vi "ParseSerializableClassHeader.vi"(8 "error in (no error)":errorcluster, 10 "Version":string[](array[string]), 11 "Class":string[](array[string])) -> (0 "error out":errorcluster, 3 "SerializedClassHeader (child,parent)":T1[](array[typedef]))   [LabVIEW 2019, in "BlueSerialization.lvlib" / "BlueSerializer.lvclass"]
uses:
  BlueSerializer.lvclass
  ClassHeader.ctl
  <vilib>/Utility/EditLVLibs/LibVersion.ctl
  <vilib>/Utility/error.llb/Error Cluster From Error Code.vi
  <vilib>/Utility/LVClass/Get LV Class Name.vi
  <vilib>/ErrorRing/Error Ring.xnode
  BlueSerializable/BlueSerializable.lvclass
  <vilib>/Utility/EditLVLibs/Edit LVLibs.lvlib
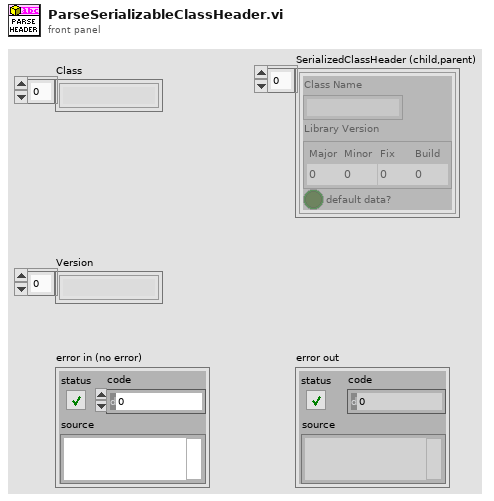
[diagram p1: front panel]
types:
  T1 = typedef "BlueSerialization.lvlib/BlueSerializer.lvclass/ClassHeader.ctl" = cluster{"Class Name":string, "Library Version":T2, "default data?":bool}
  T2 = typedef "Edit LVLibs.lvlib/LibVersion.ctl" = cluster{"Major":u16, "Minor":u16, "Fix":u16, "Build":u16}
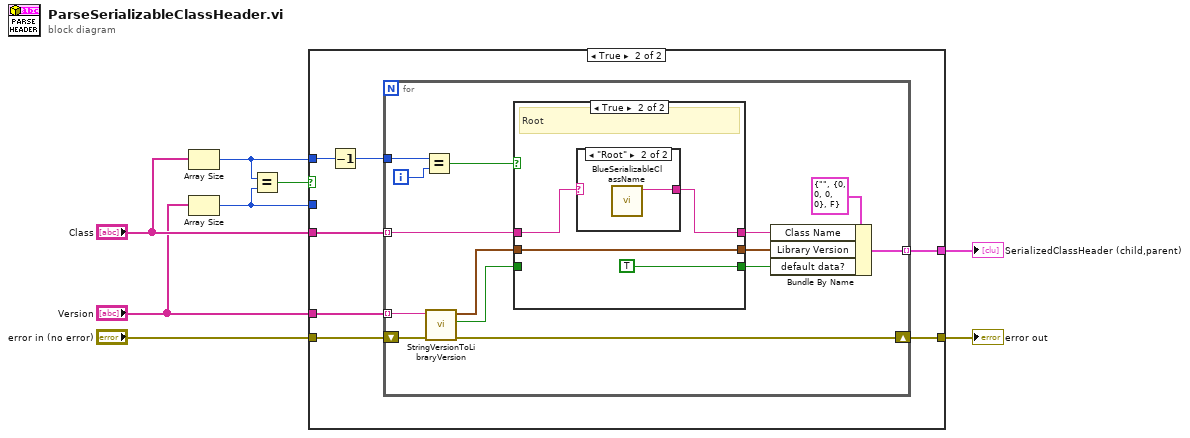
[diagram p0: block diagram]
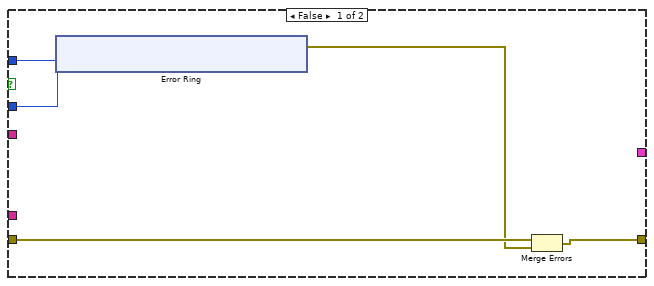
[diagram p2: hidden frame]
diagram:
  n1 = Array Size(array="Class") -> (size(s)=w3:i32)
  n2 = Array Size(array="Version") -> (size(s)=w2:i32)
  n3 = Equal?(x=w3, y=w2) -> (x = y?=w8:bool)
  n4 = case shown="True" w8 {
    tunnel: "Class" -> [_ w22]
    tunnel: "Version" -> [_ w28]
    tunnel: "error in (no error)" -> [w11 w27]
    tunnel: [w9 w26] -> w4
    tunnel: w3 -> [w13 w24]
    tunnel: w2 -> [w12 _]
    tunnel: [_ w25] -> w1
    frame False {
      n5 = xnode "Error Ring"("parameter 0"=w13, "parameter 1"=w12) -> ("error out"=w10:errorcluster)
      n6 = Merge Errors(w11, w10) -> (w9:errorcluster)
    }
    frame True {
      n7 = Decrement(x=w24) -> (x-1=w23:i32)
      n8 = for {
        tunnel: w28 -> [w41] mode=indexing
        shift-right: [w39] -> w26
        shift-left: w27 -> [w40]
        tunnel: [w38] -> w25 mode=indexing
        tunnel: w23 -> [w37]
        tunnel: w22 -> [w29] mode=indexing
        i -> [w36]
        n9 = Equal?(x=w37, y=w36) -> (x = y?=w35:bool)
        n10 = call "StringVersionToLibraryVersion.vi"("error in (no error)"=w40, "Version (as serialized)"=w41) -> ("error out"=w39:errorcluster, "default data?"=w32:bool, "Library Version"=w34:T2)  [unwired: 7 in]
        n11 = case shown="True" w35 {
          tunnel: w34 -> [w45 w47]
          tunnel: [w45 w47] -> w33
          tunnel: w32 -> [w44 _]
          tunnel: [w44 TRUE ("default data?")] -> w31
          tunnel: [w43 w48] -> w30
          tunnel: w29 -> [w43 w49]
          frame False {
            # "not root"
          }
          frame True {
            # "Root"
            n12 = case shown="\"Root\"" w49 {
              selector: w49 -> [w50 _]
              tunnel: [w50 w51] -> w48
              frame Default {
              }
              frame "Root" {
                n13 = call "BlueSerializableClassName.vi"() -> ("BlueSerialization.lvlib:BlueSerializable.lvclass"=w51:string)  [unwired: 11 in]
              }
            }
          }
        }
        n14 = Bundle By Name(cluster=T1 {"Class Name"="", "Library Version"={"Major"=0, "Minor"=0, "Fix"=0, "Build"=0}, "default data?"=FALSE} ("ClassHeader"), "Class Name"=w30, "Library Version"=w33, "default data?"=w31) -> (w38:T1)
      }
    }
  }
  "error out" <- w4
  "SerializedClassHeader (child,parent)" <- w1
